vi "update kalman COM not single cycle.vi"(10 "state in":T1) -> (2 "state out":T1)   [LabVIEW 2010]
uses:
  kalman simple pv state.ctl
  <vilib>/rvi/FXPMathLib/FxpMul/XNode/nifxpmath_Multiplier.xnode
  <vilib>/rvi/FXPMathLib/FxpMul/subVIs/nifxpmath_Mul_SimConfig.ctl
  <vilib>/fxp/LVFixedPointQuantizationPolicyTypeDef.ctl
  <vilib>/fxp/LVFixedPointOverflowPolicyTypeDef.ctl
  <vilib>/rvi/FXPMathLib/FxpDiv/XNode/nifxpmath_Div.xnode
  <vilib>/rvi/FXPMathLib/FxpDiv/subVIs/nifxpmath_Div_SimConfig.ctl
  <vilib>/rvi/FXPMathLib/FxpAdd/XNode/nifxpmath_Add.xnode
  <vilib>/rvi/FXPMathLib/FxpAdd/subVIs/nifxpmath_Add_SimConfig.ctl
  <vilib>/rvi/FXPMathLib/FxpMul/simVIs/DllFxpMulTemp_sub.vi
  <vilib>/rvi/FXPMathLib/FxpDiv/simVIs/DllFxpDivTemp_sub.vi
  <vilib>/rvi/FXPMathLib/FxpAdd/simVIs/DllFxpAddTemp_sub.vi
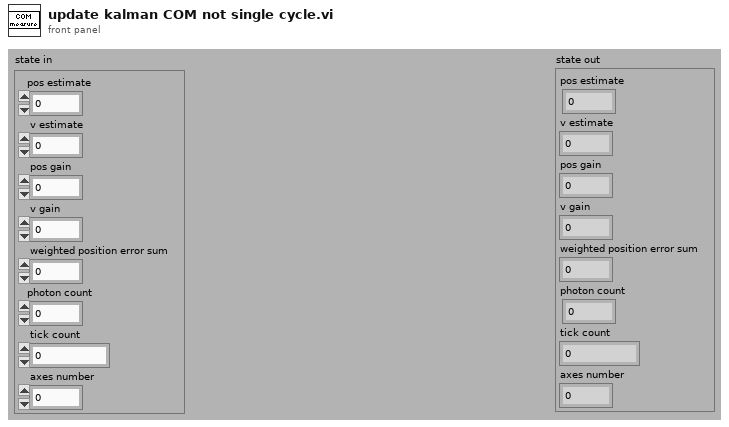
[diagram p1: front panel]
types:
  T1 = typedef "kalman simple pv state.ctl" = cluster{"pos estimate":fxp<+/-,32,16>, "v estimate":fxp<+/-,32,-4>, "pos gain":fxp<+,32,0>, "v gain":fxp<+,32,0>, "weighted position error sum":fxp<+/-,32,32>, "photon count":u32, "tick count":u32, "axes number":u8}
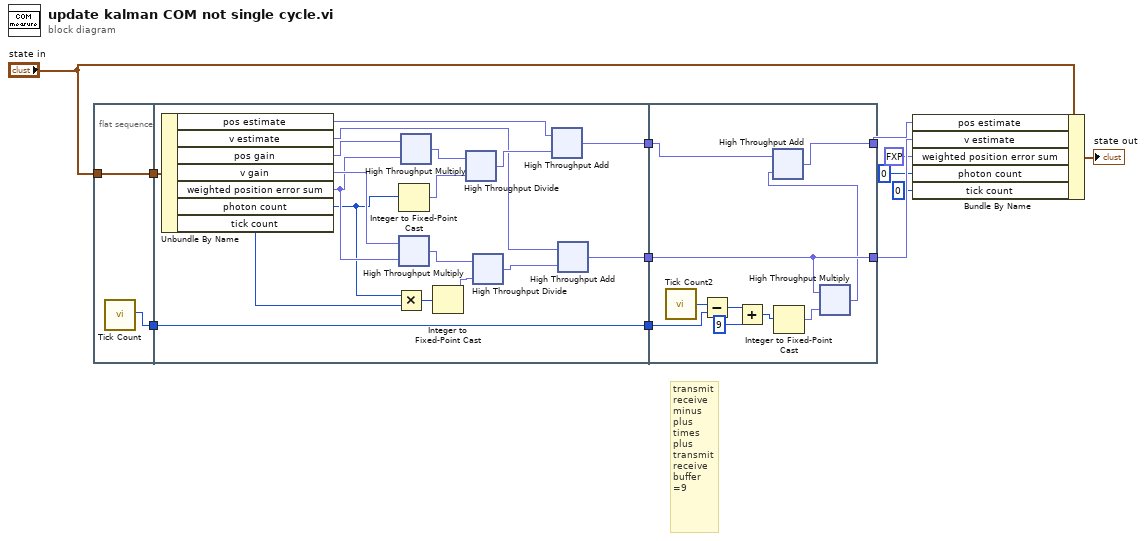
[diagram p0: block diagram]
diagram:
  # "transmit\nreceive\nminus\nplus\ntimes\nplus\ntransmit\nreceive\nbuffer\n=9"
  n1 = flat-sequence {
    tunnel: "state in" -> [w14]
    tunnel: [w14] -> w5
    tunnel: [w13] -> w2
    tunnel: w5 -> [w18]
    tunnel: [w17] -> w4
    tunnel: [w16] -> w3
    tunnel: w2 -> [w15]
    tunnel: [w15] -> w1
    tunnel: [w210] -> w10
    tunnel: [w207] -> w11
    tunnel: w4 -> [w208]
    tunnel: w3 -> [w210]
    tunnel: w1 -> [w215]
    frame #0 {
      n2 = call "Tick Count"() -> ("Tick Count(Ticks)"=w13:u16)
    }
    frame #1 {
      n3 = Unbundle By Name(w18) -> ("pos estimate"=w21:fxp<+/-,32,16>, "v estimate"=w19:fxp<+/-,32,-4>, "pos gain"=w32:fxp<+,32,0>, "v gain"=w31:fxp<+,32,0>, "weighted position error sum"=w30:fxp<+/-,32,32>, "photon count"=w26:u32, "tick count"=w25:u32)
      n4 = Multiply(x=w26, y=w25) -> (x*y=w24:u32)
      n5 = Integer to Fixed-Point Cast(integer=w26) -> (fixed-point=w28:fxp<+,32,32>)  [unwired: 1 in]
      n6 = xnode "High Throughput Multiply"("x"=w31, "y"=w30) -> ("x*y"=w27:fxp<+/-,32,32>)
      n7 = xnode "High Throughput Multiply"("x"=w32, "y"=w30) -> ("x*y"=w29:fxp<+/-,32,32>)
      n8 = Integer to Fixed-Point Cast(integer=w24) -> (fixed-point=w23:fxp<+,32,32>)  [unwired: 1 in]
      n9 = xnode "High Throughput Divide"("x"=w29, "y"=w28) -> ("x/y"=w22:fxp<+/-,32,16>)
      n10 = xnode "High Throughput Divide"("x"=w27, "y"=w23) -> ("x/y"=w20:fxp<+/-,32,-4>)
      n11 = xnode "High Throughput Add"("x"=w21, "y"=w22) -> ("x+y"=w17:fxp<+/-,32,16>)
      n12 = xnode "High Throughput Add"("x"=w19, "y"=w20) -> ("x+y"=w16:fxp<+/-,32,-4>)
    }
    frame #2 {
      n13 = call "Tick Count2"() -> ("Tick Count(Ticks)"=w216:u16)
      n14 = Subtract(x=w216, y=w215) -> (x-y=w214:u16)
      n15 = Add(x=w214, y=u16 9) -> (x+y=w212:u16)
      n16 = Integer to Fixed-Point Cast(integer=w212) -> (fixed-point=w211:fxp<+,16,16>)  [unwired: 1 in]
      n17 = xnode "High Throughput Multiply"("x"=w210, "y"=w211) -> ("x*y"=w209:fxp<+/-,32,16>)
      n18 = xnode "High Throughput Add"("x"=w208, "y"=w209) -> ("x+y"=w207:fxp<+/-,32,16>)
    }
  }
  n19 = Bundle By Name(cluster="state in", "pos estimate"=w11, "v estimate"=w10, "weighted position error sum"=fxp<+/-,32,32> 0.0, "photon count"=u32 0, "tick count"=u32 0) -> (→"state out":T1)
